vi "DSF.Engine.Sequencer.Set Iteration.vi"(8 "error in (no error)":errorcluster, 10 "iteration":u64, 11 "Sequencer Bundle in":refnum<class "Sequencer Bundle.lvclass">) -> (0 "error out":errorcluster, 3 "Sequencer Bundle out":refnum<class "Sequencer Bundle.lvclass">)   [LabVIEW 2016, in "DSF.Engine.lvlib" / "Sequencer Bundle.lvclass"]
uses:
  Sequencer Bundle.lvclass
  Sequencer Bundle.lvclass/Sequencer Bundle.ctl
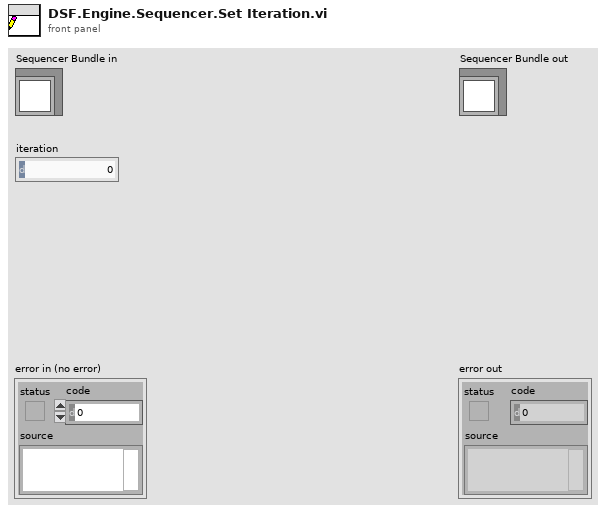
[diagram p1: front panel]
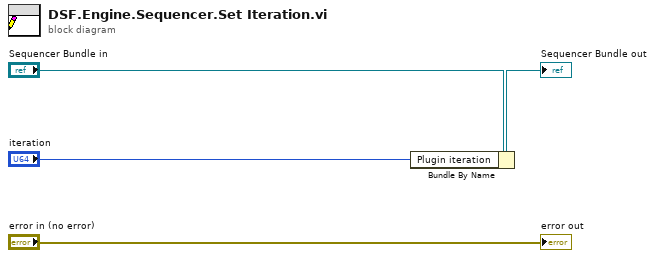
[diagram p0: block diagram]
diagram:
  n1 = Bundle By Name(cluster="Sequencer Bundle in", "Plugin iteration"="iteration") -> (→"Sequencer Bundle out":refnum<class "Sequencer Bundle.lvclass">)
  "error out" <- "error in (no error)"
